vi "Supply_SetVolts.vi"(8 "error in (no error)":errorcluster, 9 "Command string":string, 10 "Volts IN [V]":dbl, 11 "KE2657A in":refnum<class "KE2657A.lvclass">) -> (0 "error out":errorcluster, 2 "Compliance exceeded?":bool, 3 "KE2657A out":refnum<class "KE2657A.lvclass">)   [LabVIEW 2019, in "KE2657A.lvclass"]
uses:
  KE2657A.lvclass
  SupplyControl.lvclass
panel:
  out "Command sent":string
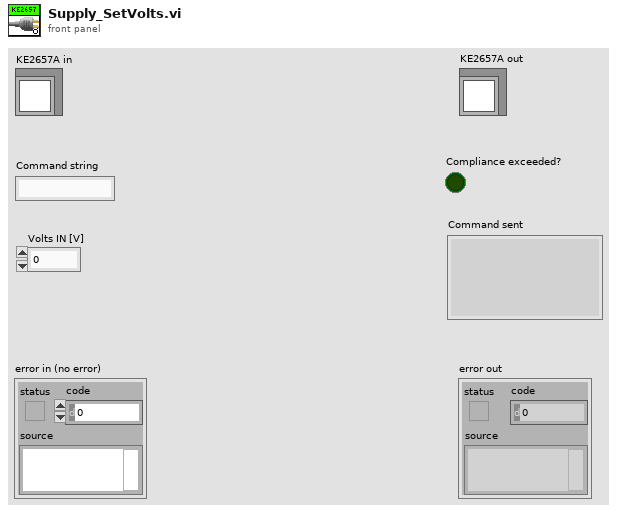
[diagram p1: front panel]
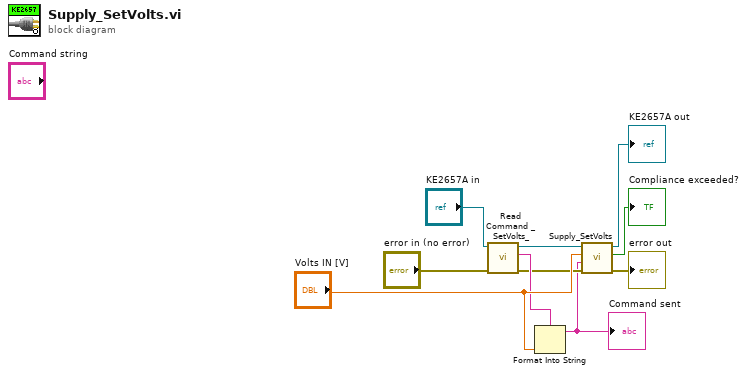
[diagram p0: block diagram]
diagram:
  n1 = call-dynamic "Read Command _SetVolts_.vi"("error in (no error)"="error in (no error)", "SupplyControl in"="KE2657A in") -> ("error out"=w3:errorcluster, "Command \"SetVolts\""=w4:string, "SupplyControl out"=w2:refnum<class "KE2657A.lvclass">)  [unwired: 7 in]
  n2 = Format Into String(format string=w4, "Volts IN [V]") -> (resulting string=w1:string)  [unwired: 2 in, 1 out]
  "Command sent" <- w1
  n3 = call-parent "Supply_SetVolts.vi"("error in (no error)"=w3, "Command string"=w1, "Volts IN [V]"="Volts IN [V]", "SupplyControl in"=w2) -> ("error out"=→"error out":errorcluster, "Compliance exceeded?"=→"Compliance exceeded?":bool, "SupplyControl out"=→"KE2657A out":refnum<class "KE2657A.lvclass">)  [unwired: 5 in]
